vi "ciacs_transforms2text.vi"(9 "A_transform":dbl[][](array[numeric]), 10 "C":dbl[](array[numeric]), 11 "B":dbl[][](array[numeric])) -> (1 "FidcucialMetrics":cluster{"M1":dbl, "M2":dbl, "S1":dbl, "S2":dbl}, 3 "Text of Transformation":string)   [LabVIEW 2011]
doc: "Create a text form of the transformation matrices and the X/Y projection scale metrics. Orthongonal scaling factors, geometric mean, and skew."
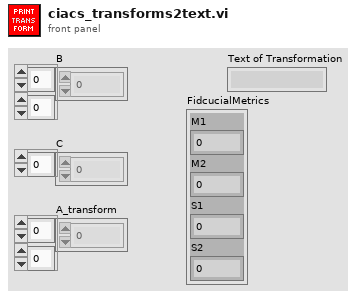
[diagram p1: front panel]
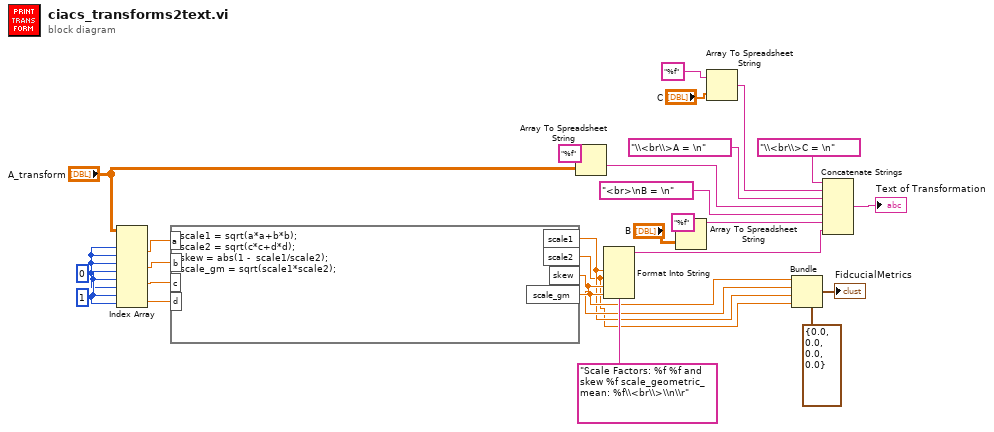
[diagram p0: block diagram]
diagram:
  w20 = 1 ("disabled index (col)")
  w19 = 0 ("index (row)")
  n1 = Index Array(array="A_transform", index (row) #1=w19, index (col) #1=w19, index (row) #2=w19, index (col) #2=w20, index (row) #3=w20, index (col) #3=w19, index (row) #4=w20, index (col) #4=w20) -> (element #1=w21:dbl, element #2=w22:dbl, element #3=w23:dbl, element #4=w24:dbl)
  n2 = formula code="scale1 = sqrt(a*a+b*b);\nscale2 = sqrt(c*c+d*d);\nskew = abs(1 -  scale1/scale2);\nscale_gm = sqrt(scale1*scale2);"("a"=w21, "b"=w22, "c"=w23, "d"=w24) -> ("scale1"=w4:dbl, "scale2"=w3:dbl, "skew"=w5:dbl, "scale_gm"=w6:dbl)
  n3 = Array To Spreadsheet String(array="A_transform", 3:"%f" ("format string")) -> (spreadsheet string=w12:string)  [unwired: 1 in]
  n4 = Format Into String(format string="Scale Factors: %f %f and skew %f scale_geometric_mean: %f\\<br\\>\\n\\r", w4, w3, w5, w6) -> (resulting string=w26:string)  [unwired: 2 in, 1 out]
  n5 = Array To Spreadsheet String(array="B", 3:"%f" ("format string")) -> (spreadsheet string=w14:string)  [unwired: 1 in]
  n6 = Array To Spreadsheet String(array="C", 3:"%f" ("format string")) -> (spreadsheet string=w10:string)  [unwired: 1 in]
  n7 = Bundle(cluster=cluster{"M1":dbl, "M2":dbl, "S1":dbl, "S2":dbl} {"M1"=0.0, "M2"=0.0, "S1"=0.0, "S2"=0.0}, "M1"=w6, "M2"=w5, "S1"=w4, "S2"=w3) -> (→"FidcucialMetrics":cluster{"M1":dbl, "M2":dbl, "S1":dbl, "S2":dbl})
  n8 = Concatenate Strings("\\<br\\>C = \n" ("string"), w10, "\\<br\\>A = \n" ("string"), w12, "<br>\nB = \n" ("string"), w14, w26) -> (→"Text of Transformation":string)
